vi "Overlay Offset Centroids.vi"(0 "Image":T1, 5 "Particle Reports (Pixels)":T2(array[cluster]), 7 "Ellipse Data":cluster{"Major":dbl, "Minor":dbl}[](array[cluster]), 9 "Bounding Rect":T3) -> (4 "Image Out":T1)   [LabVIEW 2011]
uses:
  <vilib>/vision/Image Controls.llb/IMAQ Image.ctl
  <vilib>/vision/NI_Vision_Development_Module.lvlib
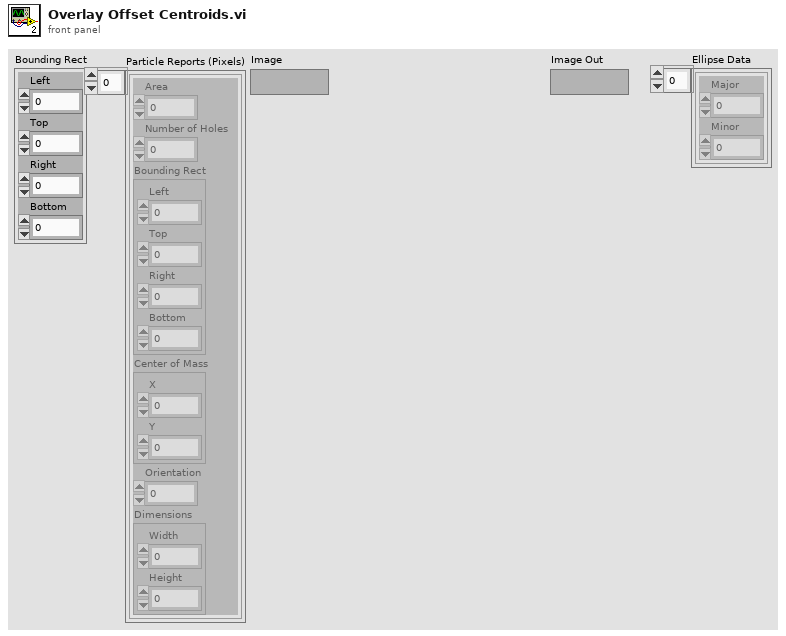
[diagram p1: front panel]
types:
  T1 = typedef "IMAQ Image.ctl" = refnum<image>
  T2 = cluster{"Area":dbl, "Number of Holes":dbl, "Bounding Rect":cluster{"Left":dbl, "Top":dbl, "Right":dbl, "Bottom":dbl}, "Center of Mass":cluster{"X":dbl, "Y":dbl}, "Orientation":dbl, "Dimensions":cluster{"Width":dbl, "Height":dbl}}[]
  T3 = cluster{"Left":dbl, "Top":dbl, "Right":dbl, "Bottom":dbl}
  T4 = typedef "Image Type" = u32
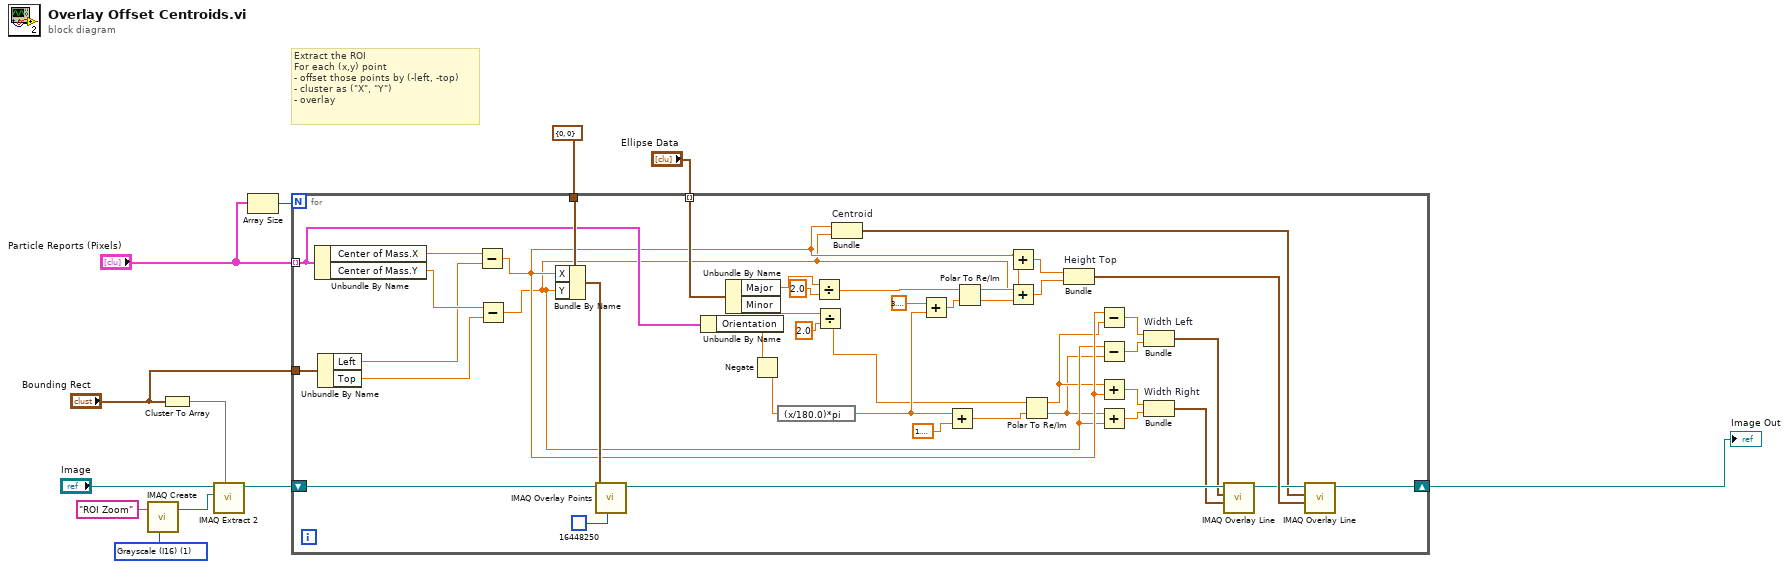
[diagram p0: block diagram]
diagram:
  w3 = T4 1 items=["Grayscale (U8)", "Grayscale (I16)", "Grayscale (SGL)", "Complex (CSG)", "RGB (U32)", "HSL (U32)", "RGB (U64)", "Grayscale (U16)"] ("Image Type")
  # "Extract the ROI\nFor each (x,y) point\n- offset those points by (-left, -top)\n- cluster as (\"X\", \"Y\")\n- overlay"
  n1 = call "IMAQ Create"("Image Name"="ROI Zoom", "Image Type"=w3) -> ("New Image"=w4:T1)  [unwired: 3 in, 1 out]
  n2 = Cluster To Array(cluster="Bounding Rect") -> (array=w8:dbl[])
  n3 = call "IMAQ Extract 2"("Optional Rectangle"=w8, "Image Dst"=w4, "Image Src"="Image") -> ("Image Dst Out"=w6:T1)  [unwired: 7 in, 1 out]
  n4 = Array Size(array="Particle Reports (Pixels)") -> (size(s)=w12:i32)
  n5 = for {
    N: w12 -> [_]
    tunnel: "Particle Reports (Pixels)" -> [w46] mode=indexing
    tunnel: cluster{"X":i32, "Y":i32} {"X"=0, "Y"=0} -> [w53]
    tunnel: "Bounding Rect" -> [w51]
    shift-right: [w40] -> w5
    shift-left: w6 -> [w48]
    tunnel: "Ellipse Data" -> [w31] mode=indexing
    n6 = Unbundle By Name(w46) -> ("Center of Mass.X"=w55:dbl, "Center of Mass.Y"=w54:dbl)
    n7 = Unbundle By Name(w51) -> ("Left"=w50:dbl, "Top"=w49:dbl)
    n8 = Subtract(x=w55, y=w50) -> (x-y=w22:dbl)
    n9 = Subtract(x=w54, y=w49) -> (x-y=w21:dbl)
    n10 = Bundle By Name(cluster=w53, "X"=w22, "Y"=w21) -> (w52:cluster{"X":i32, "Y":i32})
    n11 = call "IMAQ Overlay Points"("Color"=u32 16448250, "Point"=w52, "Image"=w48) -> ("Image Out"=w32:T1)  [unwired: 7 in, 1 out]
    n12 = Unbundle By Name(w46) -> ("Orientation"=w45:dbl)
    n13 = Unbundle By Name(w31) -> ("Major"=w30:dbl, "Minor"=w14:dbl)
    n14 = Negate(x=w45) -> (-x=w37:dbl)
    n15 = expression code="(x/180.0)*pi" ("degrees to radians")(w37) -> (w26:dbl)
    n16 = Divide(x=w30, y=2.0) -> (x/y=w29:dbl)
    n17 = Divide(x=w14, y=2.0) -> (x/y=w15:dbl)
    n18 = Bundle "Centroid"(w22, w21) -> (w24:cluster{dbl, dbl})  [unwired: 1 in]
    n19 = Add(x=3.141592653589793, y=w26) -> (x+y=w38:dbl)
    n20 = Add(x=w26, y=1.5707963267948966) -> (x+y=w27:dbl)
    n21 = Polar To Re/Im(2:w38, 3:w29) -> (0:w41:dbl, 1:w42:dbl)
    n22 = Add(x=w22, y=w42) -> (x+y=w44:dbl)
    n23 = Add(x=w21, y=w41) -> (x+y=w43:dbl)
    n24 = Polar To Re/Im(2:w27, 3:w15) -> (0:w19:dbl, 1:w20:dbl)
    n25 = Bundle "Height Top"(w44, w43) -> (w39:cluster{dbl, dbl})  [unwired: 1 in]
    n26 = Subtract(x=w22, y=w20) -> (x-y=w18:dbl)
    n27 = Subtract(x=w21, y=w19) -> (x-y=w17:dbl)
    n28 = Add(x=w20, y=w22) -> (x+y=w35:dbl)
    n29 = Add(x=w19, y=w21) -> (x+y=w34:dbl)
    n30 = Bundle "Width Left"(w18, w17) -> (w16:cluster{dbl, dbl})  [unwired: 1 in]
    n31 = Bundle "Width Right"(w35, w34) -> (w23:cluster{dbl, dbl})  [unwired: 1 in]
    n32 = call "IMAQ Overlay Line"("End Point"=w23, "Start Point"=w16, "Image"=w32) -> ("Image Out"=w33:T1)  [unwired: 7 in, 1 out]
    n33 = call "IMAQ Overlay Line"("End Point"=w39, "Start Point"=w24, "Image"=w33) -> ("Image Out"=w40:T1)  [unwired: 7 in, 1 out]
  }
  "Image Out" <- w5
